vi "RunCommVi.vi"(8 "error in (no error)":errorcluster, 11 "Client.lvclass in":refnum<class "Client.lvclass">) -> (0 "error out":errorcluster, 3 "Client.lvclass out":refnum<class "Client.lvclass">)   [LabVIEW 2018, in "Client.lvclass"]
uses:
  Client.lvclass
  Client.lvclass/Client.ctl
  Comm/Stream/Stream.lvclass
panel:
  out "error out 2":errorcluster
  out "error out 3":errorcluster
  out "error out 5":errorcluster
  out "error out 4":errorcluster
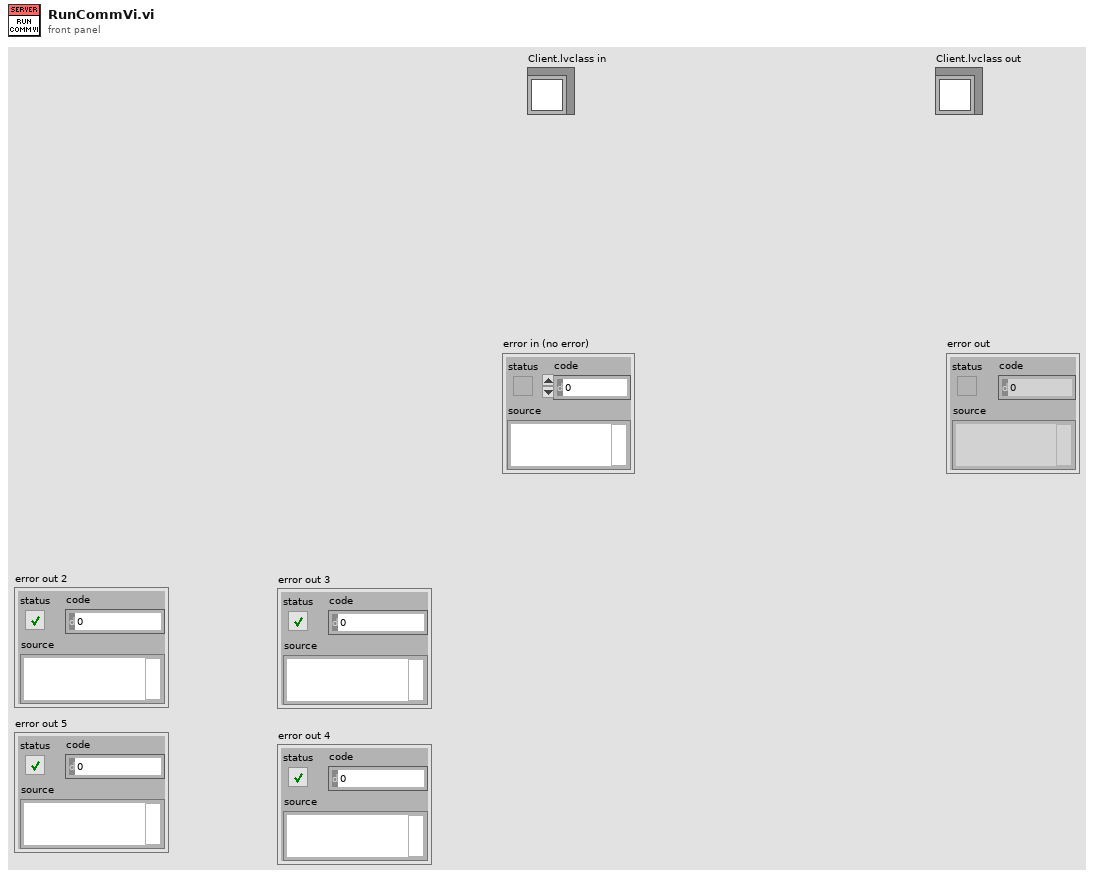
[diagram p1: front panel]
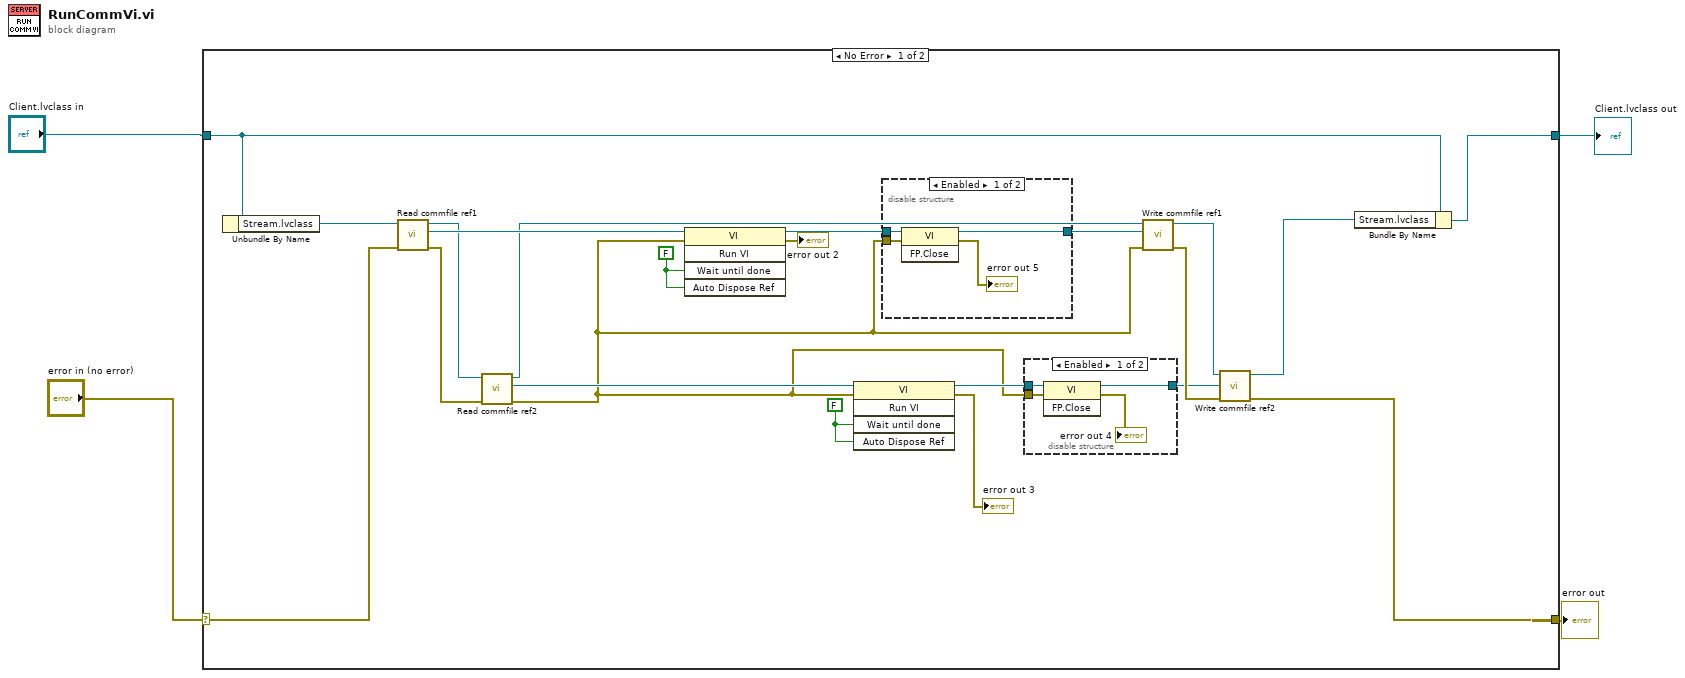
[diagram p0: block diagram]
diagram:
  n1 = case shown="No Error" "error in (no error)" {
    selector: "error in (no error)" -> [w21 w38]
    tunnel: [w17 w38] -> w3
    tunnel: [w26 w37] -> w2
    tunnel: "Client.lvclass in" -> [w25 w37]
    frame No Error {
      w12 = FALSE ("Wait Until Done")
      w13 = FALSE ("Wait Until Done")
      n2 = Unbundle By Name(w25) -> ("Stream.lvclass"=w24:refnum<class "Stream.lvclass">)
      n3 = call-dynamic "Read commfile ref1.vi"("error in (no error)"=w21, "Stream in"=w24) -> ("error out"=w20:errorcluster, "commfile ref1"=w23:refnum<vi>, "Stream out"=w16:refnum<class "Stream.lvclass">)  [unwired: 7 in]
      n4 = call-dynamic "Read commfile ref2.vi"("error in (no error)"=w20, "Stream in"=w16) -> ("error out"=w6:errorcluster, "commfile ref2"=w22:refnum<vi>, "Stream out"=w19:refnum<class "Stream.lvclass">)  [unwired: 7 in]
      n5 = invoke class="VI" method="Run VI"(reference=w23, error in=w6, "Wait until done"=w13, "Auto Dispose Ref"=w13) -> (reference out=w7:refnum<vi>, error out=→"error out 2":errorcluster)  [unwired: 1 in, 3 out]
      n6 = invoke class="VI" method="Run VI"(reference=w22, error in=w6, "Wait until done"=w12, "Auto Dispose Ref"=w12) -> (reference out=w9:refnum<vi>, error out=→"error out 3":errorcluster)  [unwired: 1 in, 3 out]
      n7 = disable-structure shown="Enabled" {
        disable-tunnel: w7 -> [w35 w36]
        disable-tunnel: w6 -> [w34 _]
        disable-tunnel: [w32 w36] -> w5
        frame Enabled {
          n8 = invoke class="VI" method="FP.Close"(reference=w35, error in=w34) -> (reference out=w32:refnum<vi>, error out=→"error out 5":errorcluster)  [unwired: 1 in, 1 out]
        }
        frame Disabled {
        }
      }
      n9 = disable-structure shown="Enabled" {
        disable-tunnel: w9 -> [w30 w31]
        disable-tunnel: [w29 w31] -> w8
        disable-tunnel: w6 -> [w27 _]
        frame Enabled {
          n10 = invoke class="VI" method="FP.Close"(reference=w30, error in=w27) -> (reference out=w29:refnum<vi>, error out=→"error out 4":errorcluster)  [unwired: 1 in, 1 out]
        }
        frame Disabled {
        }
      }
      n11 = call-dynamic "Write commfile ref1.vi"("error in (no error)"=w6, "commfile ref1"=w5, "Stream in"=w19) -> ("error out"=w18:errorcluster, "Stream out"=w15:refnum<class "Stream.lvclass">)  [unwired: 7 in]
      n12 = call-dynamic "Write commfile ref2.vi"("error in (no error)"=w18, "commfile ref2"=w8, "Stream in"=w15) -> ("error out"=w17:errorcluster, "Stream out"=w14:refnum<class "Stream.lvclass">)  [unwired: 7 in]
      n13 = Bundle By Name(cluster=w25, "Stream.lvclass"=w14) -> (w26:refnum<class "Client.lvclass">)
    }
    frame Error {
    }
  }
  "error out" <- w3
  "Client.lvclass out" <- w2
